vi "Write T start stop.vi"(8 "error in (no error)":errorcluster, 11 "Heater in":refnum<class "Heater.lvclass">) -> (0 "error out":errorcluster, 3 "Heater out":refnum<class "Heater.lvclass">)   [LabVIEW 2019, in "Heating.lvlib" / "Heater.lvclass"]
uses:
  Heater.lvclass
  Heater.lvclass/Heater.ctl
  REG/HE_reg.lvclass/HE_reg.ctl
  Reg/PID/PID SP Limiter/PID SP Limiter.lvclass/PID SP Limiter.ctl
  HE_state.lvclass/HE_state.ctl
  ZM_state/HE_ZM_state.lvclass/HE_ZM_state.ctl
  Reg/PID/PID SP Limiter/PID SP Limiter.lvclass
  ZM_state/HE_ZM_state.lvclass
  REG/HE_reg.lvclass
  HE_state.lvclass
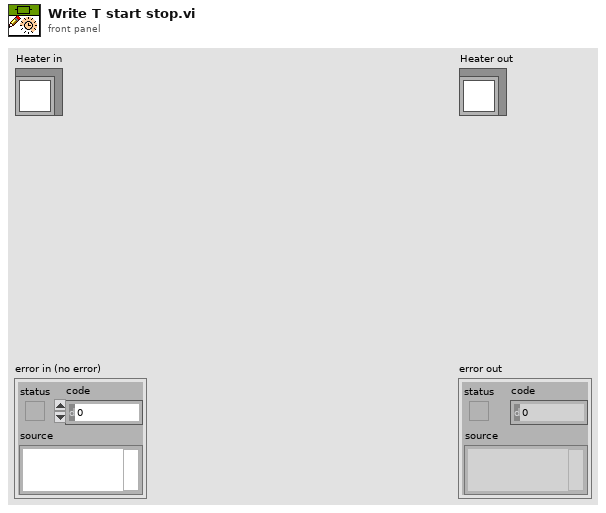
[diagram p1: front panel]
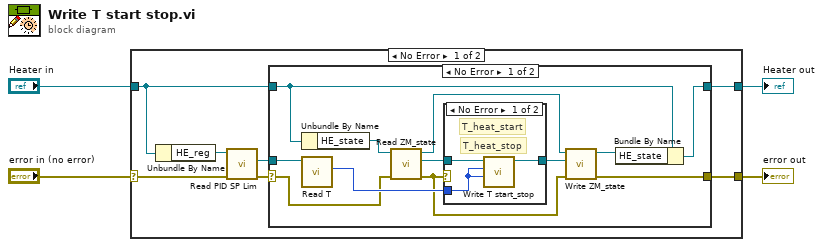
[diagram p0: block diagram]
diagram:
  n1 = case shown="No Error" "error in (no error)" {
    selector: "error in (no error)" -> [w7 w31]
    tunnel: [w9 w31] -> w3
    tunnel: [w10 w30] -> w1
    tunnel: "Heater in" -> [w11 w30]
    frame No Error {
      n2 = Unbundle By Name(w11) -> ("HE_reg"=w8:refnum<class "HE_reg.lvclass">)
      n3 = call "Read PID SP Lim.vi"("error in (no error)"=w7, "HE_reg in"=w8) -> ("error out"=w6:errorcluster, "PID SP Limiter"=w5:refnum<class "PID SP Limiter.lvclass">)  [unwired: 7 in, 1 out]
      n4 = case shown="No Error" w6 {
        selector: w6 -> [w18 w28]
        tunnel: w5 -> [w23 _]
        tunnel: w11 -> [w21 w29]
        tunnel: [w20 w29] -> w10
        tunnel: [w13 w28] -> w9
        frame No Error {
          n5 = Unbundle By Name(w21) -> ("HE_state"=w19:refnum<class "HE_state.lvclass">)
          n6 = call "Read T.vi"("PID SP Limiter in"=w23) -> ("T"=w22:u32)  [unwired: 9 in, 1 out]
          n7 = call "Read ZM_state.vi"("error in (no error)"=w18, "HE_state in"=w19) -> ("error out"=w12:errorcluster, "HE_ZM_state"=w17:refnum<class "HE_ZM_state.lvclass">, "HE_state out"=w16:refnum<class "HE_state.lvclass">)  [unwired: 7 in]
          n8 = case shown="No Error" w12 {
            tunnel: w17 -> [w26 w27]
            tunnel: w22 -> [w24 _]
            tunnel: [w25 w27] -> w15
            frame No Error {
              # "T_heat_stop"
              # "T_heat_start"
              n9 = call "Write T start_stop.vi"("T_heat_stop"=w24, "T_heat_start"=w24, "HE_ZM_state in"=w26) -> ("HE_ZM_state out"=w25:refnum<class "HE_ZM_state.lvclass">)  [unwired: 8 in]
            }
            frame Error {
            }
          }
          n10 = call "Write ZM_state.vi"("error in (no error)"=w12, "HE_ZM_state"=w15, "HE_state in"=w16) -> ("error out"=w13:errorcluster, "HE_state out"=w14:refnum<class "HE_state.lvclass">)  [unwired: 7 in]
          n11 = Bundle By Name(cluster=w21, "HE_state"=w14) -> (w20:refnum<class "Heater.lvclass">)
        }
        frame Error {
        }
      }
    }
    frame Error {
    }
  }
  "error out" <- w3
  "Heater out" <- w1
